vi "_keysight_generate_pulses.vi"(0 "Ch1 pulse_width (ns)":dbl=100.0, 1 "Ch2 pulse_width (ns)":dbl=20.0, 2 "Ch1 pulse_delay (ns)":dbl=20.0, 3 "Ch2 pulse_delay (ns)":dbl, 4 "error in":errorcluster) -> (5 "Command":string=":pulse:width1 100.000NS\n:pulse:width2 20.000NS\n:pulse:delay1 20.000NS\n:pulse:delay2 0.000NS", 6 "error out":errorcluster)   [LabVIEW 2013]
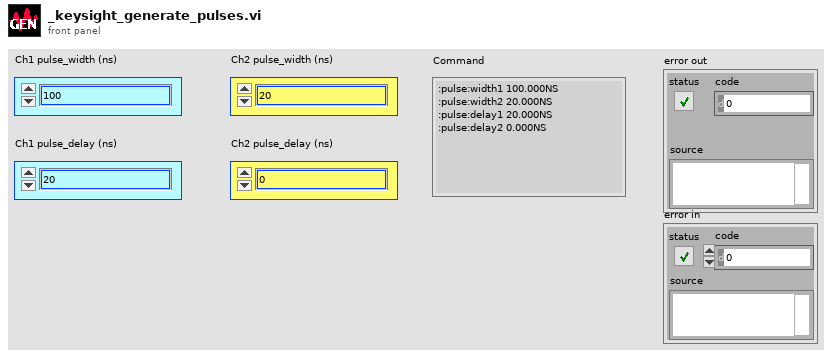
[diagram p1: front panel]
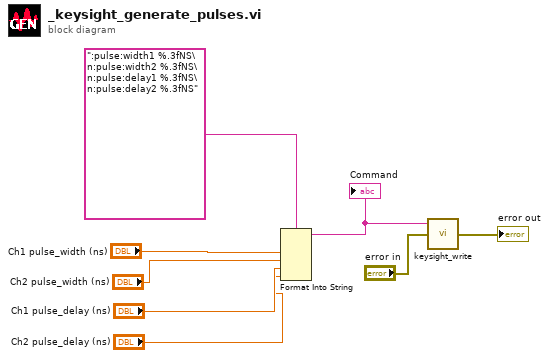
[diagram p0: block diagram]
diagram:
  n1 = Format Into String(format string=":pulse:width1 %.3fNS\n:pulse:width2 %.3fNS\n:pulse:delay1 %.3fNS\n:pulse:delay2 %.3fNS", "Ch1 pulse_width (ns)", "Ch2 pulse_width (ns)", "Ch1 pulse_delay (ns)", "Ch2 pulse_delay (ns)") -> (resulting string=w6:string)  [unwired: 2 in, 1 out]
  "Command" <- w6
  n2 = call "keysight_write.vi"("error in"="error in", "command"=w6) -> ("error out"=→"error out":errorcluster)  [unwired: 1 in]
